vi "Configure System Trigger.vi"(7 "Timer Interval (0.1 s)":dbl=0.1, 8 "error in (no error)":errorcluster, 9 "Control Source (0: Immediate)":i32(ring) items=["Immediate", "Manual", "Bus", "External", "Timer"], 10 "Trigger Mode (0: Continuous)":i32(ring) items=["Continuous", "One-shot"], 11 "VISA resource name":refnum<visa-resource-name>) -> (0 "error out":errorcluster, 3 "VISA resource name out":refnum<visa-resource-name>)   [LabVIEW 2016, in "Keithley 6517.lvlib"]
doc: "Configures settings for system trigger.\n\n<B>Note:</B>\nThis VI is <B>NOT</B> compatible with model <B>6514</B>."
uses:
  <instrlib>/Keithley 6517/Keithley 6517.lvlib
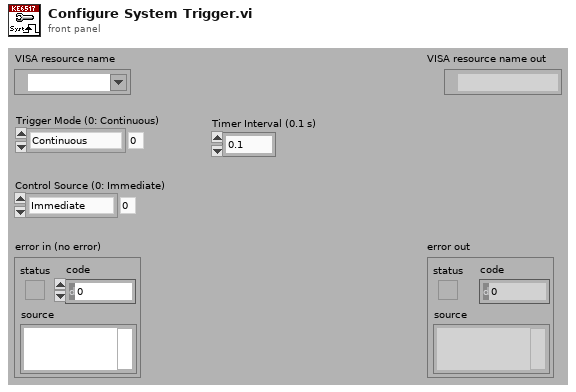
[diagram p1: front panel]
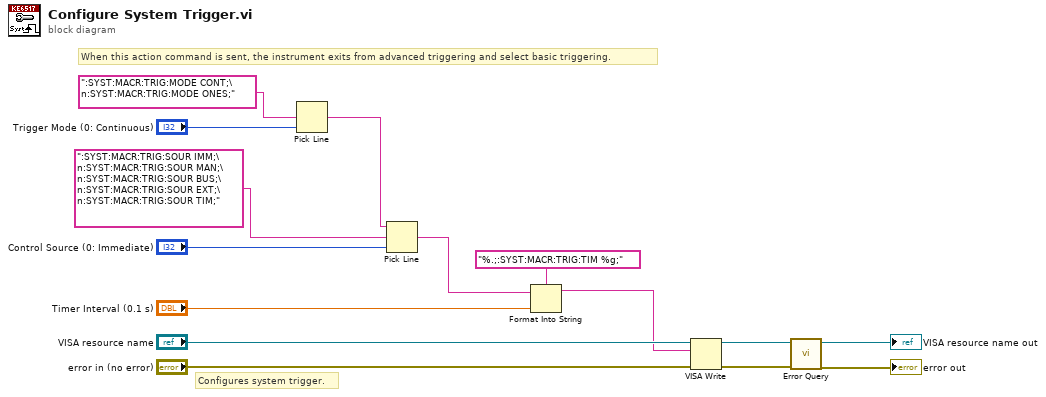
[diagram p0: block diagram]
diagram:
  # "When this action command is sent, the instrument exits from advanced triggering and select basic triggering."
  # "Configures system trigger."
  n1 = Pick Line(multi-line string=":SYST:MACR:TRIG:MODE CONT;\n:SYST:MACR:TRIG:MODE ONES;", line index="Trigger Mode (0: Continuous)") -> (output string=w3:string)  [unwired: 1 in]
  n2 = Pick Line(string ("")=w3, multi-line string=":SYST:MACR:TRIG:SOUR IMM;\n:SYST:MACR:TRIG:SOUR MAN;\n:SYST:MACR:TRIG:SOUR BUS;\n:SYST:MACR:TRIG:SOUR EXT;\n:SYST:MACR:TRIG:SOUR TIM;", line index="Control Source (0: Immediate)") -> (output string=w2:string)
  n3 = Format Into String(format string="%.;:SYST:MACR:TRIG:TIM %g;", initial string=w2, "Timer Interval (0.1 s)") -> (resulting string=w8:string)  [unwired: 1 in, 1 out]
  n4 = VISA Write(VISA resource name="VISA resource name", write buffer=w8, error in (no error)="error in (no error)") -> (VISA resource name out=w12:refnum<visa-resource-name>, error out=w11:errorcluster)  [unwired: 1 out]
  n5 = call <instrlib>:"Error Query.vi"("error in (no error)"=w11, "VISA resource name"=w12) -> ("error out"=→"error out":errorcluster, "VISA resource name out"=→"VISA resource name out":refnum<visa-resource-name>)  [unwired: 6 in, 2 out]
